vi "sub_multipart.vi"() -> ()   [LabVIEW 2014]
uses:
  lvnanomsg/socket_type.ctl
  lvnanomsg/nanomsg.lvlib
  lvnanomsg/nanomsg_context.lvclass
  lvnanomsg/nanomsg_socket.lvclass
panel:
  out "message":string[](array[string])
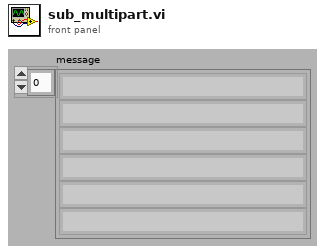
[diagram p1: front panel]
types:
  T1 = enum16{"NN_SUB_XXX", "NN_SUB_SUBSCRIBE", "NN_SUB_UNSUBSCRIBE"}
  T2 = typedef "nanomsg.lvlib/socket_type.ctl" = enum8{"NN_SOL_SOCKET", "NN_1", "NN_2", "NN_3", "NN_4", "NN_5", "NN_6", "NN_7", "NN_8", "NN_9", "NN_10", "NN_11", "NN_12", "NN_13", "NN_14", "NN_15", "NN_PAIR", "NN_17", "NN_18", "NN_19", "NN_20", "NN_21", "NN_22", "NN_23", "NN_24", "NN_25", "NN_26", "NN_27", "NN_28", "NN_29", "NN_30", "NN_31", "NN_PUB", "NN_SUB", "NN_34", "NN_35", "NN_36", "NN_37", "NN_38", "NN_39", "NN_40", "NN_41", "NN_42", "NN_43", "NN_44", "NN_45", "NN_46", "NN_47", "REQ_REQ", "REP_REP", "NN_50", "NN_51", "NN_52", "NN_53", "NN_54", "NN_55", "NN_56", "NN_57", "NN_58", "NN_59", "NN_60", "NN_61", "NN_62", "NN_63", "NN_64", "NN_65", "NN_66", "NN_67", "NN_68", "NN_69", "NN_70", "NN_71", "NN_72", "NN_73", "NN_74", "NN_75", "NN_76", "NN_77", "NN_78", "NN_79", "NN_PUSH", "NN_PULL", "NN_82", "NN_83", "NN_84", "NN_85", "NN_86", "NN_87", "NN_88", "NN_89", "NN_90", "NN_91", "NN_92", "NN_93", "NN_94", "NN_95", "NN_96", "NN_97", "NN_SURVEYOR", "NN_RESPONDENT", "NN_100", "NN_101", "NN_102", "NN_103", "NN_104", "NN_105", "NN_106", "NN_107", "NN_108", "NN_109", "NN_110", "NN_111", "NN_BUS"}
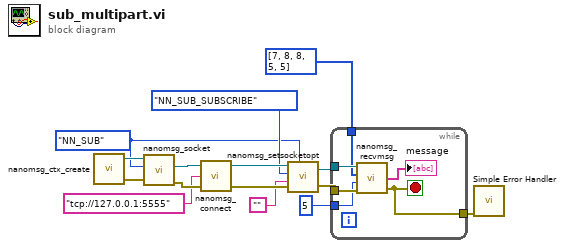
[diagram p0: block diagram]
diagram:
  w3 = socket_type."NN_SUB" ("socket type")
  n1 = call "nanomsg_ctx_create.vi"() -> ("error out"=w15:errorcluster, "context out"=w4:refnum<class "nanomsg_context.lvclass">)  [unwired: 4 in]
  n2 = call "nanomsg_socket.vi"("error in"=w15, "socket type"=w3, "context in"=w4) -> ("error out"=w14:errorcluster, "socket out"=w5:refnum<class "nanomsg_socket.lvclass">)  [unwired: 2 in, 1 out]
  n3 = call "nanomsg_connect.vi"("error in"=w14, "endpoint"="tcp://127.0.0.1:5555", "socket in"=w5) -> ("error out"=w12:errorcluster, "socket out"=w13:refnum<class "nanomsg_socket.lvclass">)  [unwired: 1 in]
  n4 = call "nanomsg_setsocketopt.vi"("socket in"=w13, "option"=T1."NN_SUB_SUBSCRIBE", "value"="", "error in"=w12, "level"=w3) -> ("socket out"=w10:refnum<class "nanomsg_socket.lvclass">, "error out"=w11:errorcluster)
  n5 = while {
    tunnel: w10 -> [w21]
    tunnel: w11 -> [w19]
    tunnel: [w18] -> w6
    tunnel: 5 -> [w17]
    tunnel: i32[] [7, 8, 8, 5, 5] -> [w16]
    stop <- w18 stop-if-true
    n6 = call "nanomsg_recvmsg.vi"("socket in"=w21, "lenvec"=w16, "size"=w17, "error in"=w19) -> ("parts"=→"message":string[], "error out"=w18:errorcluster)  [unwired: 1 in, 1 out]
  }
  n7 = call <vilib>:"Simple Error Handler.vi"("error in (no error)"=w6) -> ()  [unwired: 4 in, 5 out]
